vi "EOL Oscope AI Current Buffer.vi"(8 "Data to Write (Ch-Ro, Samp-Col)":sgl[][](array[numeric]) format="%.2f", 9 "Buffer Size (seconds/2500)":i32=5000, 11 "Mode":T1(ring)=enum."Read") -> (2 "Data Read (Ch-Ro, Samp-Col)":sgl[][](array[numeric]) format="%.2f")   [LabVIEW 2018]
doc: "This VI is used in many locations throughout the program as a data buffer. It serves mainly two purposes. In alarms and logging, the DAQ data, whether scaled or voltage, is entered into the buffer. In other parts of the program, data is read from the buffer. Its length is based on the # of samples it was initialized to.\n\nA read will always return the latest data of the size requested."
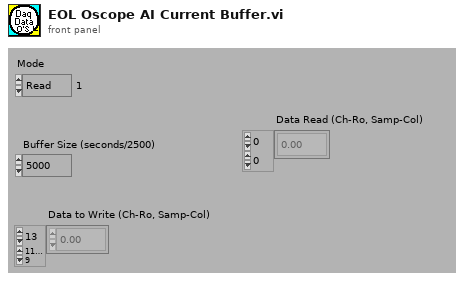
[diagram p1: front panel]
types:
  T1 = enum16{"Initialize", "Read", "Write", "Read other"}
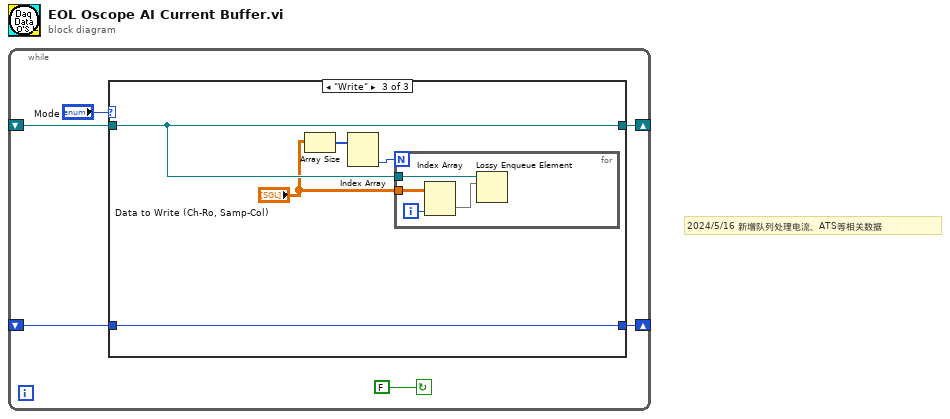
[diagram p0: block diagram]
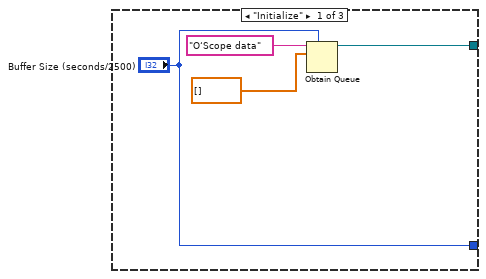
[diagram p2: hidden frame]
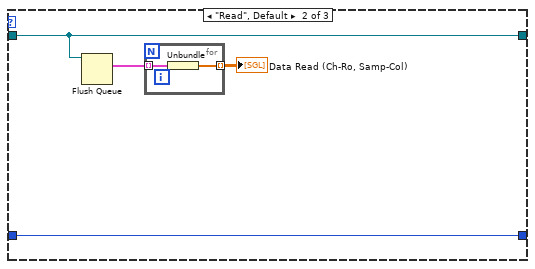
[diagram p3: hidden frame]
diagram:
  # "2024/5/16 新增队列处理电流、ATS等相关数据"
  n1 = while {
    shift-left: _ -> [w5]
    shift-right: [w4] -> _
    shift-right: [w2] -> _
    shift-left: _ -> [w1]
    stop <- FALSE continue-if-true
    n2 = case shown="\"Write\"" "Mode" {
      tunnel: ["Buffer Size (seconds/2500)" w14 w21] -> w4
      tunnel: w5 -> [_ w14 w21]
      tunnel: [w9 w13 w20] -> w2
      tunnel: w1 -> [_ w13 w20]
      frame "Initialize" {
        n3 = Obtain Queue(max queue size (-1, unlimited)="Buffer Size (seconds/2500)", name (unnamed)="O‘Scope data" ("名称"), element data type=sgl[] []) -> (queue out=w9:refnum<queue>)  [unwired: 2 in, 2 out]
      }
      frame "Read", Default {
        n4 = Flush Queue(queue=w13) -> (remaining elements=w12:cluster{sgl[]}[])  [unwired: 1 in, 2 out]
        n5 = for {
          tunnel: w12 -> [w16] mode=indexing
          tunnel: [w15] -> w11 mode=indexing
          n6 = Unbundle(w16) -> (w15:sgl[])
        }
        "Data Read (Ch-Ro, Samp-Col)" <- w11
      }
      frame "Write" {
        n7 = Array Size(array="Data to Write (Ch-Ro, Samp-Col)") -> (size(s)=w19:i32[])
        n8 = Index Array(array=w19) -> (element #2=w18:i32)  [unwired: 2 in, 1 out]
        n9 = for {
          N: w18 -> [_]
          tunnel: w20 -> [w25]
          tunnel: "Data to Write (Ch-Ro, Samp-Col)" -> [w24]
          i -> [w22]
          n10 = Index Array(array=w24, index (col)=w22) -> (element=w23:sgl[])  [unwired: 1 in]
          n11 = Lossy Enqueue Element(queue=w25, element=w23) -> ()  [unwired: 1 in, 4 out]
        }
      }
    }
  }
